vi "loadConfig.vi"(8 "error in (no error)":errorcluster caption="错误输入（无错误）", 10 "calFilePath":string, 11 "5071C 输入":refnum<class "5071C.lvclass"> caption="DNL_LabVIEW Object in") -> (0 "error out":errorcluster caption="错误输出", 3 "5071C 输出":refnum<class "5071C.lvclass"> caption="DNL_LabVIEW Object out")   [LabVIEW 2011, in "5071C.lvclass"]
uses:
  5071C.lvclass
  5071C.lvclass/5071C.ctl
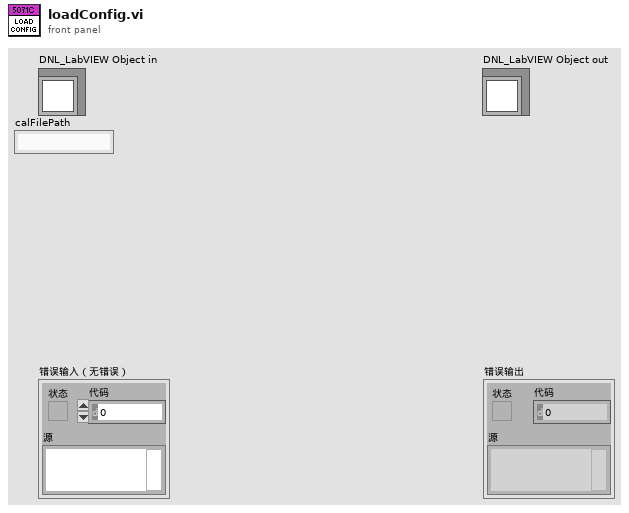
[diagram p1: front panel]
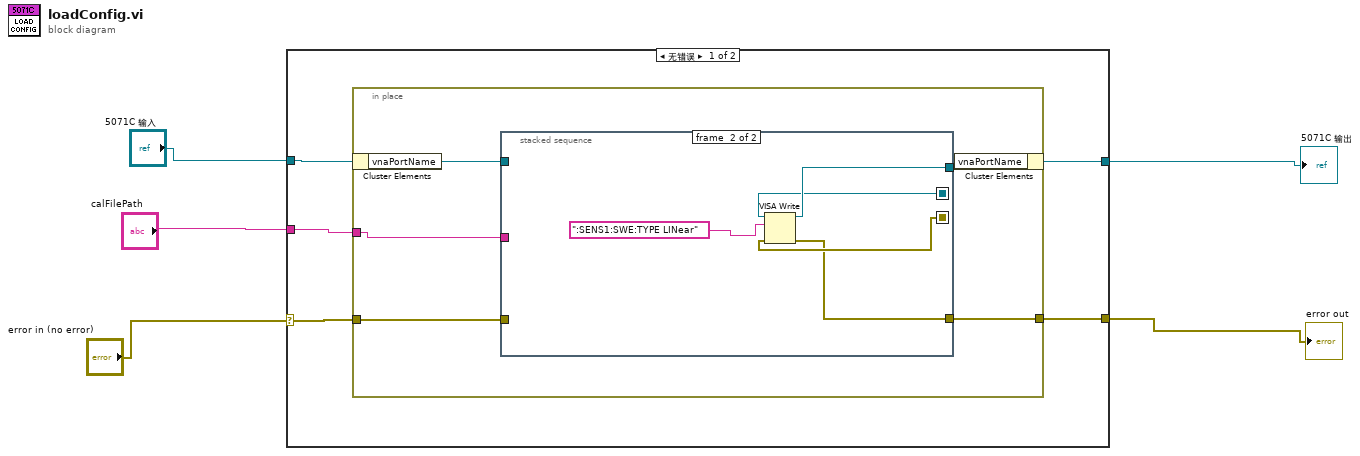
[diagram p0: block diagram]
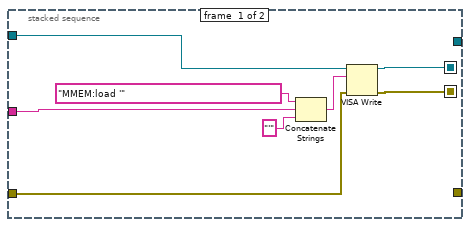
[diagram p2: hidden frame]
diagram:
  n1 = case shown="无错误" "error in (no error)" {
    selector: "error in (no error)" -> [w7 w30]
    tunnel: "5071C 输入" -> [w10 w29]
    tunnel: "calFilePath" -> [w9 _]
    tunnel: [w8 w29] -> w4
    tunnel: [w6 w30] -> w2
    frame No Error {
      n2 = in-place {
        in-place-border: w9 -> [w14]
        in-place-border: w7 -> [w12]
        in-place-border: [w11] -> w6
        n3 = in-place-cluster #1(w10) -> ("vnaPortName"=w15:refnum<visa-resource-name>)
        n4 = stacked-sequence {
          seq-local: [w17 _] -> [_ w27]
          seq-local: [w16 _] -> [_ w26]
          tunnel: w15 -> [w23 _]
          tunnel: w14 -> [w19 _]
          tunnel: [_ w28] -> w13
          tunnel: w12 -> [w18 _]
          tunnel: [_ w25] -> w11
          frame #0 {
            n5 = Concatenate Strings("MMEM:load '" ("write buffer"), w19, "'" ("字符串")) -> (w21:string)
            n6 = VISA Write(VISA resource name=w23, write buffer=w21, error in (no error)=w18) -> (VISA resource name out=w17:refnum<visa-resource-name>, error out=w16:errorcluster)  [unwired: 1 out]
          }
          frame #1 {
            n7 = VISA Write(VISA resource name=w27, write buffer=":SENS1:SWE:TYPE LINear", error in (no error)=w26) -> (VISA resource name out=w28:refnum<visa-resource-name>, error out=w25:errorcluster)  [unwired: 1 out]
          }
        }
        n8 = in-place-cluster #1("vnaPortName"=w13) -> (w8:refnum<class "5071C.lvclass">)
      }
    }
    frame Error {
    }
  }
  "error out" <- w2
  "5071C 输出" <- w4
